vi "Variables.vi"() -> ()   [LabVIEW 2013]
panel:
  in  "Contrôle des boucles":bool
  out "Graphe déroulant 2":dbl(graph)
  out "Graphe déroulant 1":dbl(graph)
  # "Off"
  # "On"
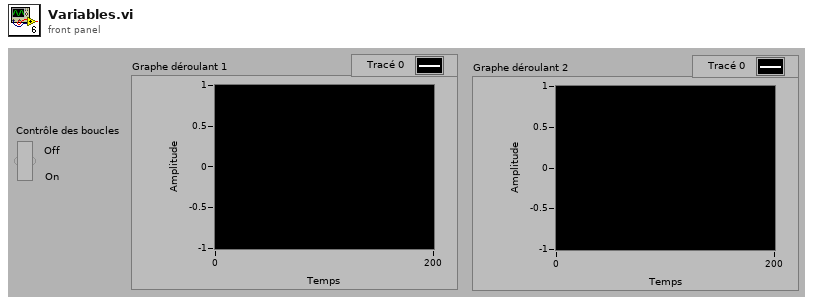
[diagram p1: front panel]
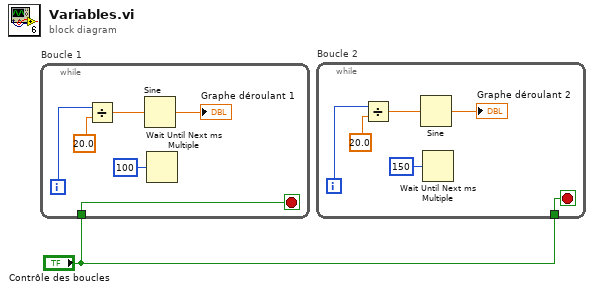
[diagram p0: block diagram]
diagram:
  n1 = while "Boucle 1" {
    tunnel: "Contrôle des boucles" -> [w2]
    i -> [w7]
    stop <- w2 stop-if-true
    n2 = Divide ("Diviser")(x=w7, y=20.0) -> (x/y=w5:dbl)
    n3 = Sine ("Sinus")(x=w5) -> (sin(x)=→"Graphe déroulant 1":dbl)
    n4 = Wait Until Next ms Multiple ("Attendre un multiple de ms")(millisecond multiple=u32 100) -> ()  [unwired: 1 out]
  }
  n5 = while "Boucle 2" {
    tunnel: "Contrôle des boucles" -> [w8]
    i -> [w13]
    stop <- w8 stop-if-true
    n6 = Divide ("Diviser")(x=w13, y=20.0) -> (x/y=w11:dbl)
    n7 = Sine ("Sinus")(x=w11) -> (sin(x)=→"Graphe déroulant 2":dbl)
    n8 = Wait Until Next ms Multiple ("Attendre un multiple de ms")(millisecond multiple=u32 150) -> ()  [unwired: 1 out]
  }
